vi "JOG LIMIT.vi"(8 "error in (no error)":errorcluster, 11 "main ref":T1) -> (0 "error out":errorcluster)   [LabVIEW 2025]
uses:
  controls/LAB-IQ UI Data.ctl
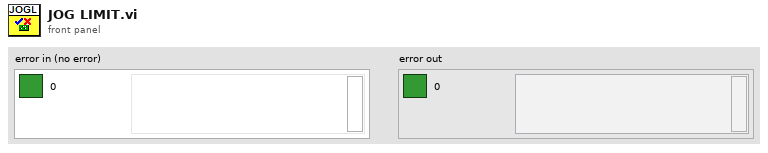
[diagram p1: front panel]
types:
  T1 = typedef "LAB-IQ UI Data.ctl" = cluster{"Main Home Screen":cluster{"GUI":refnum<vi>, "Platform Settings":refnum<vi>, "Configure":refnum<vi>, "Home":refnum<vi>, "EXIT":refnum<vi>, "service 2":refnum<vi>, "MainPage":refnum<vi>, "Analysis":refnum<vi>}, "Platform Settings":cluster{"mm/s  Surge":refnum<vi>, "Update Surge Speed":refnum<vi>, "Drive Error":refnum<vi>, "Disable Axis Jog Soft Limits":refnum<vi>, "mm/s  Sway":refnum<vi>, "Sway and Surge COM Status":refnum<vi>, "Heave COM Status":refnum<vi>, "Enable Platform":refnum<vi>, "Surge Forward Main":refnum<vi>, "Sway Right Main":refnum<vi>, "Sway Left Main":refnum<vi>, "Heave Down Main":refnum<vi>, "Heave Up main":refnum<vi>, "Update Sway Speed":refnum<vi>, "Update Heave Speed":refnum<vi>, "mm/s Heave":refnum<vi>, "mm/sec":refnum<vi>, "mm":refnum<vi>, "Surge Backward Main":refnum<vi>}, "Analysis Screen":cluster{"Analysis Home":refnum<vi>, "Surface Analysis":refnum<vi>, "Imaging":refnum<vi>, "Image Analysis":refnum<vi>, "Post Analysis":refnum<vi>}, "Config Screen":cluster{"Select Load Head":refnum<vi>, "Notes :":refnum<vi>, "FILE":refnum<vi>, "Sample ID :":refnum<vi>, "Operator ID :":refnum<vi>, "Operator Name :":refnum<vi>, "Auto":refnum<vi>}, "Motion Module":cluster{"zNL":refnum<vi>, "NL disp":refnum<vi>, "Rotary Tab":refnum<vi>, "Motion Direction:  3":refnum<vi>, "E.Velocity 2":refnum<vi>, "e.v/ssr 2":refnum<vi>, "Enter Fixed E.Velocity 2":refnum<vi>, "Enter Final SRR 2":refnum<vi>, "Enter initial SRR 2":refnum<vi>, "Enter Fixed SRR 2":refnum<vi>, "Enter the Final E.Velocity (m/s) 2":refnum<vi>, "Enter initial E.Velocity (m/s) 2":refnum<vi>, "Final Speed (RPM) 3":refnum<vi>, "Initial Speed (RPM) 2":refnum<vi>, "Enter the Final Velocity (m/s) 3":refnum<vi>, "Enter initial Velocity (m/s)  3":refnum<vi>, "Ramp Up 2":refnum<vi>, "TEST SELECTION":refnum<vi>, "SPEED SELECTION : ":refnum<vi>, "Angular Oscillation Set":refnum<vi>, "Traction":refnum<vi>, "Step Speed":refnum<vi>, "StepTable For Load-Speed":refnum<vi>, "StepTable For Speed":refnum<vi>, "Surge Forward MM":refnum<vi>, "Surge Backward MM":refnum<vi>, "M3 Image":refnum<vi>, "String 39":refnum<vi>, "Sway Left MM":refnum<vi>, "Sway Right MM":refnum<vi>, "Disable Axis Jog Soft Limits":refnum<vi>, "mm":refnum<vi>, "Heave Down MM":refnum<vi>, "Heave Up MM":refnum<vi>, "Wear Track Diameter (mm)":refnum<vi>, "Set WTD":refnum<vi>, "HomeScratch":refnum<vi>, "HomeRot":refnum<vi>, "PlaceModule":refnum<vi>, "Enter the Angle (Deg)":refnum<vi>, "Enter the Frequency (Hz)":refnum<vi>, "Motion Mode:":refnum<vi>, "LR Sway":refnum<vi>, "Rot Hor":refnum<vi>, "Scratch":refnum<vi>, "LR Cam":refnum<vi>, "MMBack":refnum<vi>, "MMNext":refnum<vi>, "Rot Ver":refnum<vi>, "Rotary Module Selection":refnum<vi>, "calculate rotary":refnum<vi>, "SPEED SELECTION : rotary":refnum<vi>, "Import 2":refnum<vi>, "Save 2":refnum<vi>, "File Path :  2":refnum<vi>, "String 45":refnum<vi>, "StepTable For Speed 3":refnum<vi>, "Enter the Speed(mm/sec)":refnum<vi>, "Enter the Speed(RPM)":refnum<vi>, "Enter Scratch Speed (mm/s):":refnum<vi>, "SwaySpeed Set":refnum<vi>, "Scartch Offset":refnum<vi>, "Motion type:":refnum<vi>, "HomeScratch 2":refnum<vi>, "Enter Scratch length (mm):":refnum<vi>, "Wear Track Diameter":refnum<vi>, "Rotary Speed Exced":refnum<vi>, "Scratch Mode":refnum<vi>, "No of Scratch":refnum<vi>}, "Environmental control":cluster{"Humidity  Status  3":refnum<vi>, "Low Temp  Status  2":refnum<vi>, "TK4 status 2":refnum<vi>, "Stage Temperature":refnum<vi>, "Sample Temperature":refnum<vi>, "Humidity (Amb)":refnum<vi>, "Clear List":refnum<vi>, "Add to list":refnum<vi>, "Wear":refnum<vi>, "Vibration":refnum<vi>, "Humidity (Chamber)":refnum<vi>, "Temperature (Chamber)":refnum<vi>, "ECR ":refnum<vi>, "Temperature (Amb)":refnum<vi>, "Microphone":refnum<vi>, "Acoustic Emission 3":refnum<vi>, "SNext":refnum<vi>, "APBack":refnum<vi>, "Enter the Temperature (°C):":refnum<vi>, "Enter the Stage \nTemperature (°C):":refnum<vi>, "Enter the Humidity (%Rh):":refnum<vi>, "Low Temp":refnum<vi>, "High Temp":refnum<vi>, "Humidity":refnum<vi>, "Sensors Picked":refnum<vi>}, "About Screen":cluster{"Password":refnum<vi>, "Home Service":refnum<vi>, "Advanced Setting":refnum<vi>, "About Tab":refnum<vi>, "ECR Port:":refnum<vi>, "Ramp Port:":refnum<vi>, "Installation/Replacement completed":refnum<vi>, "Loahead":refnum<vi>, "Heave and Surge COM Port:":refnum<vi>, "Sway COM Port:":refnum<vi>, "Temp Modbus:":refnum<vi>, "Humidity Port:":refnum<vi>, "Edit Gain Constants":refnum<vi>, "Save Gain Constants":refnum<vi>}, "Main Screen":cluster{"Main Screen Tab":refnum<vi>, "Angle and Frequency":refnum<vi>, "Stroke (mm)":refnum<vi>, "Angle (Deg)":refnum<vi>, "Main Speed Tab":refnum<vi>, "MTM MOTOR DISPLAY":refnum<vi>, "Disc Speed (m/sec)":refnum<vi>, "Ball Speed (m/sec)":refnum<vi>, "Disc Speed (RPM)":refnum<vi>, "Ball Speed (RPM)":refnum<vi>, "SPEED TAB":refnum<vi>, "Speed (m/sec)":refnum<vi>, "Set Speed (m/sec)":refnum<vi>, "Speed (RPM)":refnum<vi>, "Set Speed":refnum<vi>, "Time Tab":refnum<vi>, "Time ( HH:MM:SS ) 2":refnum<vi>, "Test Duration":refnum<vi>, "Test Duration 4":refnum<vi>, "TEST CYCLE":refnum<vi>, "TOTAL CYCLES":refnum<vi>, "Set Load (N)":refnum<vi>, "Temp Tabs":refnum<vi>, "Heater":refnum<vi>, "TK4 status":refnum<vi>, "ChamberTemp":refnum<vi>, "SetTmp":refnum<vi>, "Controller  Status":refnum<vi>, "ChamberTemp 2":refnum<vi>, "SetTmp 2":refnum<vi>, "Controller  Status 2":refnum<vi>, "ChamberTemp 3":refnum<vi>, "SetTmp 3":refnum<vi>, "Cooling":refnum<vi>, "Load Communication":refnum<vi>, "Ambient \nTemperature":refnum<vi>, "HumCOMStatus":refnum<vi>, "Ambient\n Humidity":refnum<vi>, "Freq (Hz)":refnum<vi>, "Load En":refnum<vi>, "NLt":refnum<vi>, "zNL 2":refnum<vi>, "Humidity On":refnum<vi>, "humidity disp":refnum<vi>, "Set Humidity":refnum<vi>, "NL disp 2":refnum<vi>, "Humidity On 2":refnum<vi>, "humidity disp 2":refnum<vi>, "Set Humidity 2":refnum<vi>, "NL disp 3":refnum<vi>, "AppLoadSeq scratch":refnum<vi>, "Stop Scratch":refnum<vi>, "ClrLog":refnum<vi>, "Trip Log":refnum<vi>, "STOP":refnum<vi>, "Start Test":refnum<vi>, "Test status":refnum<vi>, "AR Led":refnum<vi>, "Data":refnum<vi>, "Health":refnum<vi>, "Sway COM Status":refnum<vi>, "Heave COM Status":refnum<vi>, "Grp Tab":refnum<vi>, "Sub Graph":refnum<vi>, "SD (mm)":refnum<vi>, "Siliding distance Reset Graph":refnum<vi>, "SDGp":refnum<vi>, "Humidity Reset Graph":refnum<vi>, "HumrGp":refnum<vi>, "Acoustic Emission (mV)":refnum<vi>, "Aqucostic Reset Graph":refnum<vi>, "gACQUOS":refnum<vi>, "ECR RESET":refnum<vi>, "ECR":refnum<vi>, "Temperature Reset":refnum<vi>, "Acoustic Emission (mV) 2":refnum<vi>, "Aqucostic Reset Graph 2":refnum<vi>, "gACQUOS 2":refnum<vi>, "ECR RESET 2":refnum<vi>, "ECR 2":refnum<vi>, "Temperature Reset 2":refnum<vi>, "Temperature (deg c)":refnum<vi>, "Speed Reset Graph":refnum<vi>, "Speed Tab":refnum<vi>, "MTM DISC  SPEED":refnum<vi>, "MTM BALL SPEED":refnum<vi>, "speed mm/sec":refnum<vi>, "Hymidity":refnum<vi>, "Humidity Disable trip":refnum<vi>, "CoF Trip  2":refnum<vi>, "Depth Trip":refnum<vi>, "Weart Deapth":refnum<vi>, "Depth Reset Graph":refnum<vi>, "Weart":refnum<vi>, "Depthz":refnum<vi>, "Depth (µm)":refnum<vi>, "WearGp":refnum<vi>, "NL Trip 2":refnum<vi>, "Load pid":refnum<vi>, "Load Disable Trip":refnum<vi>, "Load Reset Graph":refnum<vi>, "NL Display 4":refnum<vi>, "Main Chart 3":refnum<vi>, "BACK":refnum<vi>, "Depth Trip 2":refnum<vi>, "COF TRIP ":refnum<vi>, "Friction Force (N)":refnum<vi>, "FF Reset Graph":refnum<vi>, "FF Disable Trip":refnum<vi>, "FF TRIP":refnum<vi>, "COF Disable Trip":refnum<vi>, "COF Reset Graph":refnum<vi>, "Start Test Temp":refnum<vi>, "zFF":refnum<vi>, "Friction Force (N) Graph":refnum<vi>, "Coefficient of Friction":refnum<vi>, "Scratch Start Test":refnum<vi>, "FF Tab":refnum<vi>, "Cyclic Friction Force (N)":refnum<vi>, "CZ FF":refnum<vi>, "Cyclic Friction Force (N) Graph":refnum<vi>, "Cyclic Coefficient of Friction":refnum<vi>, "Cyclic FF TRIP":refnum<vi>, "Cyclic FF Disable Trip":refnum<vi>, "cyclic COF Disable Trip":refnum<vi>, "cyclic COF TRIP":refnum<vi>, "cyclic COF Reset Graph":refnum<vi>, "Cyclic FF Reset Graph":refnum<vi>, "Test Trip":refnum<vi>, "Multi Scratch Pass":refnum<vi>, "Scratch Start Recording":refnum<vi>}, "Loading":cluster{"Indentation":refnum<vi>, "Reference Sample":refnum<vi>, "Load Cell Communication Slide":refnum<vi>, "com 3":refnum<vi>, "com":refnum<vi>, "DecaForce COM Status":refnum<vi>, "Update":refnum<vi>, "Clear 3":refnum<vi>, "seq":refnum<vi>, "Stribeck table":refnum<vi>, "Stribeck Table  For loading":refnum<vi>, "Loading Mode":refnum<vi>, "Enter the Final Load (N)":refnum<vi>, "Enter the CoF Trip":refnum<vi>, "Enter the Friction Force Trip":refnum<vi>, "Enter the Normal load Trip":refnum<vi>, "Enter the Load  (N)":refnum<vi>, "KiloForce":refnum<vi>, "DecaForce ":refnum<vi>, "MicroForce":refnum<vi>, "LHBack":refnum<vi>, "LHNext":refnum<vi>, "Enter the Loading Rate (N/min)":refnum<vi>, "Message":refnum<vi>, "Warning 2":refnum<vi>, "SSP 0.75":refnum<vi>, "SSP 0.5":refnum<vi>, "SSP 0.3":refnum<vi>, "Warning":refnum<vi>, "gui GIF":refnum<vi>, "Communication is established":refnum<vi>, "AppLoad 4":refnum<vi>, "Multipoint":refnum<vi>, "Load Selection":refnum<vi>}, "PID":cluster{"Ramp MulFac":refnum<vi>, "pulses LoadDiffRamp(2..10)":refnum<vi>, "PulseControlRamp(diff<=3N)":refnum<vi>, "SetLoadDeadband(%) Load(0-10N)":refnum<vi>, "PID gains out delay (microForce)":refnum<vi>, "Ramp":refnum<vi>, "Gain 2":refnum<vi>, "pulses LoadDiff(2..10)":refnum<vi>, "pulses LoadDiff(11..50)":refnum<vi>, "PulseControl(diff<=3N)":refnum<vi>, "SetLoadDeadband(%)  2":refnum<vi>, "Dummy Run":refnum<vi>, "Vertical load (N)":refnum<vi>, "AutoTune":refnum<vi>, "Offset 3 ":refnum<vi>, "apply load":refnum<vi>, "Offset  3":refnum<vi>, "apply load 2":refnum<vi>, "Enter ByPass Load":refnum<vi>, "reinit 3":refnum<vi>, "output range delay":refnum<vi>, "PID gains out delay":refnum<vi>, "Bypass Load":refnum<vi>, "pulsesSent":refnum<vi>, "pulses ":refnum<vi>, "actpid":refnum<vi>, "gFF Rot":refnum<vi>, "pulses LoadDiff(21..1000)":refnum<vi>, "Delay":refnum<vi>, "deadband":refnum<vi>}, "Config Parameters":cluster{"Tab Control 3":refnum<vi>, "Tab Control 19":refnum<vi>, "SAMPLES":refnum<vi>, "Re-initilaize":refnum<vi>, "Filter ON/OFF":refnum<vi>, "TracHomeSurgeOffsetCounts 10MM":refnum<vi>, "TracHomeSwayOffsetCounts 10MM":refnum<vi>, "Acoustic Emission:":refnum<vi>, "Apply Filter (FF)":refnum<vi>, "Filter% 2":refnum<vi>, "Apply Filter (Load)":refnum<vi>, "Filter% ":refnum<vi>, "Sway distance (mm)":refnum<vi>, "Surge distance (mm)":refnum<vi>, "DataSavingLoopDelay(ms)":refnum<vi>, "SAVE 2":refnum<vi>, "Enter Distance":refnum<vi>, "Sway Counts:":refnum<vi>, "Distance (mm): 3":refnum<vi>, "Surge Counts:":refnum<vi>, "Distance (mm): 2":refnum<vi>, "Distance (mm):":refnum<vi>, "Heave Counts:":refnum<vi>, "LRMHomeSurgeOffsetCounts":refnum<vi>, "LRMHomeSwayOffsetCounts":refnum<vi>, "TracHomeSurgeOffsetCounts 20MM":refnum<vi>, "TracHomeSwayOffsetCounts 20MM":refnum<vi>, "RotHomeSwayOffsetCounts":refnum<vi>, "RotHomeSurgeOffsetCounts":refnum<vi>, "Heave distance":refnum<vi>, "Zmm":refnum<vi>, "Heave Pulses/mm":refnum<vi>, "Surge Pulses/mm":refnum<vi>, "Sway Pulses/mm":refnum<vi>, "Heave Pitch":refnum<vi>, "Surge Pitch":refnum<vi>, "Sway Pitch":refnum<vi>, "Heave PPR":refnum<vi>, "Surge PPR":refnum<vi>, "Sway PPR":refnum<vi>, "Tab Control 5":refnum<vi>, "Tab Control 14":refnum<vi>, "Tab Control 26":refnum<vi>, "AE":refnum<vi>, "Heave Loop Delay":refnum<vi>, "Heave PID Speed":refnum<vi>, "Surge Jog Speed":refnum<vi>, "Heave Jog Speed":refnum<vi>, "Sway Loop Delay":refnum<vi>, "Sway PID Speed":refnum<vi>, "Sway Jog Speed":refnum<vi>, "DEPTH TRIP VALUE":refnum<vi>, "LOAD TRIP VALUE":refnum<vi>, "DEPTH TRIP   ENABLE":refnum<vi>, "LOAD TRIP  ENABLE":refnum<vi>, "CYCLIC FF TRIP VALUE":refnum<vi>, "FF TRIP VALUE":refnum<vi>, "CYCLIC CoF TRIP VALUE":refnum<vi>, "COF TRIP VALUE":refnum<vi>, "CYCLIC COF TRIP  ENABLE":refnum<vi>, "CYCLIC FF TRIP  ENABLE":refnum<vi>, "FF TRIP  ENABLE":refnum<vi>, "COF TRIP  ENABLE":refnum<vi>}, "Loading Com Port":cluster{"ClearAll":refnum<vi>, "Mz(Nm)":refnum<vi>, "My(Nm)":refnum<vi>, "Mx(Nm)":refnum<vi>, "Save Dwell":refnum<vi>, "Mx ":refnum<vi>, "My ":refnum<vi>, "Mz":refnum<vi>, "Fx(N)":refnum<vi>, "Fy(N)":refnum<vi>, "Fz(N)":refnum<vi>, "ZeroAll":refnum<vi>, "Acq Delay (ms)":refnum<vi>, "Burst Delay (ms)":refnum<vi>, "model":refnum<vi>, "SN":refnum<vi>, "FFx(N)":refnum<vi>, "Sensor IP":refnum<vi>, "Port":refnum<vi>, "FFy(N)":refnum<vi>, "Load(N)":refnum<vi>, "delete Handle":refnum<vi>, "Create Handle":refnum<vi>, "ft_data":refnum<vi>, "ft_range":refnum<vi>, "ft_data 2":refnum<vi>, "stop 6":refnum<vi>, "running_flag":refnum<vi>, "ft_udp_handle":refnum<vi>, "get-data-return":refnum<vi>, "get-range-return":refnum<vi>, "zero-return":refnum<vi>, "filter-return":refnum<vi>, "initial-return":refnum<vi>, "deleteHandle-result":refnum<vi>, "Load Cell Temp":refnum<vi>}, "Heave AND Surge":cluster{"SURGE POSE":refnum<vi>, "error out Read":refnum<vi>, "HEAVE POSE":refnum<vi>, "State":refnum<vi>, "Homed":refnum<vi>, "Sequence ID":refnum<vi>, "error out Write":refnum<vi>, "faultCode":refnum<vi>, "Ack ID":refnum<vi>, "SPEED":refnum<vi>, "Distance":refnum<vi>, "Mode Command":refnum<vi>, "Heave and Surge Read":refnum<vi>, "Read Heave Temp":refnum<vi>, "Spare 15":refnum<vi>, "Spare 14":refnum<vi>, "Spare 13":refnum<vi>, "Spare 12":refnum<vi>, "Spare 11":refnum<vi>, "Spare 10":refnum<vi>, "Spare 9":refnum<vi>, "Spare 8":refnum<vi>, "Spare 7":refnum<vi>, "Spare 6":refnum<vi>, "Spare 5":refnum<vi>, "Spare 4":refnum<vi>, "Spare 2":refnum<vi>, "Spare 1":refnum<vi>, "Node Id":refnum<vi>, "Spare 3":refnum<vi>, "SPARE 4":refnum<vi>, "SPARE 3":refnum<vi>, "SPARE 2":refnum<vi>, "SPARE 1":refnum<vi>, "fwMajor":refnum<vi>, "fwMinor":refnum<vi>, "Manual Write":refnum<vi>, "Heave and Surge Write":refnum<vi>}, "New PID LOGIC":cluster{"Fine Tune Zone":refnum<vi>, "PID SDelay":refnum<vi>, "Max_pos_limit":refnum<vi>, "Min_pos_limit":refnum<vi>, "i_limit":refnum<vi>, "pct_scale":refnum<vi>, "Deadband":refnum<vi>, "Kd":refnum<vi>, "Ki":refnum<vi>, "Kp":refnum<vi>, "Current Position":refnum<vi>, "Set Load":refnum<vi>, "Current Load":refnum<vi>, "Pulse delta":refnum<vi>, "Init Step":refnum<vi>, "Max Step Linit":refnum<vi>}, "SWAY ":cluster{"fwMajor":refnum<vi>, "Homed":refnum<vi>, "Rotary POSE":refnum<vi>, "State":refnum<vi>, "SWAY POSE":refnum<vi>, "Ack ID":refnum<vi>, "faultCode":refnum<vi>, "Node Id":refnum<vi>, "fwMinor":refnum<vi>, "Spare 6":refnum<vi>, "Spare 5":refnum<vi>, "Spare 4":refnum<vi>, "Spare 3":refnum<vi>, "Spare 2":refnum<vi>, "Spare 1":refnum<vi>, "Spare 7":refnum<vi>, "SPARE  5":refnum<vi>, "error out Write  SWAY ":refnum<vi>, "error out Read SWAY ":refnum<vi>, "Manual Write SWAY ":refnum<vi>, "SWAY WRITE":refnum<vi>, "SPARE  4":refnum<vi>, "SPARE  3":refnum<vi>, "SPARE 2":refnum<vi>, "SPARE 1":refnum<vi>, "Spare 15":refnum<vi>, "Spare 14":refnum<vi>, "Spare 13":refnum<vi>, "Spare 12":refnum<vi>, "Spare 11":refnum<vi>, "Spare 9":refnum<vi>, "Spare 8":refnum<vi>, "SPEED":refnum<vi>, "Distance":refnum<vi>, "Mode Command":refnum<vi>, "Sequence ID":refnum<vi>, "SWAY READ":refnum<vi>, "Spare 10":refnum<vi>, "Read SWAY Temp":refnum<vi>}, "Analysis Screen":cluster{"Analysis Home":refnum<vi>, "Refresh 2":refnum<vi>, "MEAN 4":refnum<vi>, "SD 4":refnum<vi>, "VARIANCE 4":refnum<vi>, "MEAN  3":refnum<vi>, "SD  3":refnum<vi>, "VARIANCE  3":refnum<vi>, "MEAN 2":refnum<vi>, "SD  2":refnum<vi>, "VARIANCE 2":refnum<vi>, "MEAN":refnum<vi>, "SD":refnum<vi>, "VARIANCE":refnum<vi>, "File 4 Discription":refnum<vi>, "OPEN 4":refnum<vi>, "File Name 4":refnum<vi>, "OPEN 3":refnum<vi>, "File 3 Discription":refnum<vi>, "File Name 3":refnum<vi>, "Y-AXIS":refnum<vi>, "X-AXIS":refnum<vi>, "XY Graph":refnum<vi>, "File Name 2":refnum<vi>, "File Name 1":refnum<vi>, "OPEN 2":refnum<vi>, "OPEN 1":refnum<vi>, "File 1 Discription ":refnum<vi>, "File 2 Discription":refnum<vi>, "Export":refnum<vi>, "File Format":refnum<vi>}}
  T2 = enum8{"Enabled", "Disabled", "Disabled and Grayed Out"}
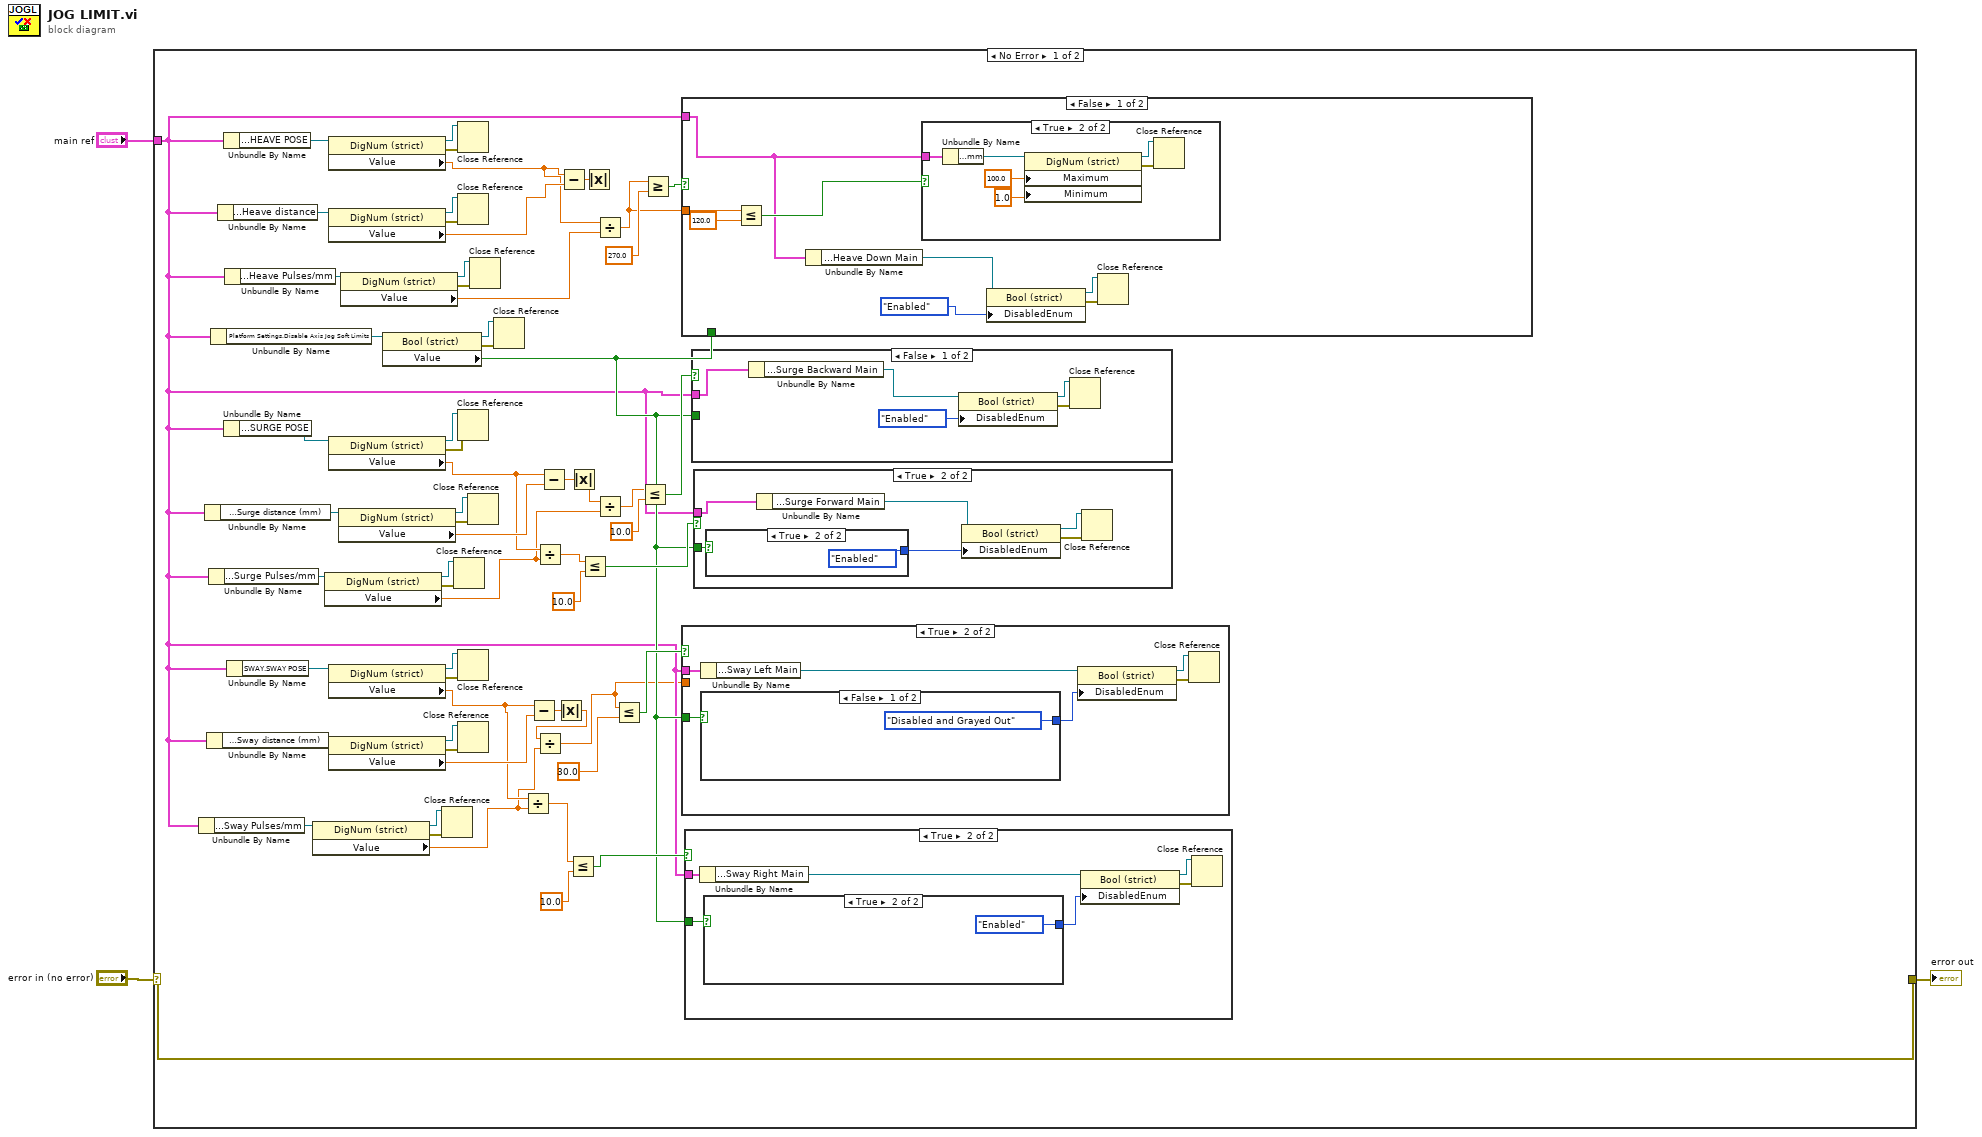
[diagram p0: block diagram]
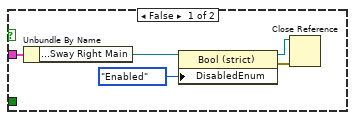
[diagram p2: hidden frame]
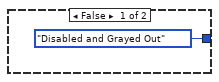
[diagram p3: hidden frame]
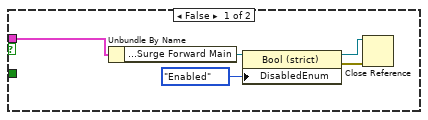
[diagram p4: hidden frame]
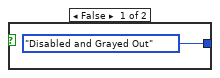
[diagram p5: hidden frame]
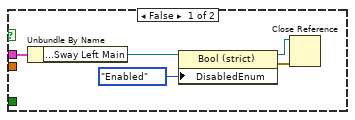
[diagram p6: hidden frame]
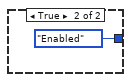
[diagram p7: hidden frame]
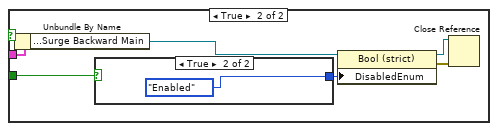
[diagram p8: hidden frame]
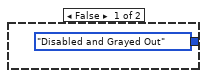
[diagram p9: hidden frame]
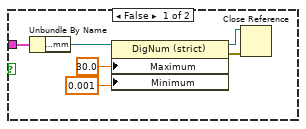
[diagram p10: hidden frame]
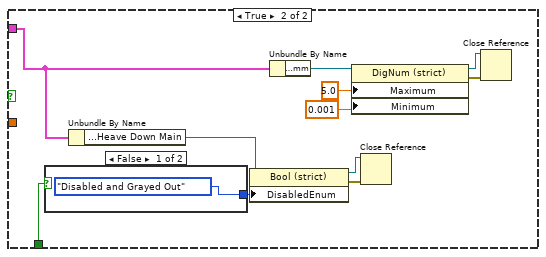
[diagram p11: hidden frame]
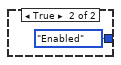
[diagram p12: hidden frame]
diagram:
  n1 = case shown="No Error" "error in (no error)" {
    selector: "error in (no error)" -> [w65 _]
    tunnel: [w65 _] -> w2
    tunnel: "main ref" -> [w13 _]
    frame No Error {
      n2 = Unbundle By Name(w13) -> ("Config Parameters.Sway Pulses/mm"=w28:refnum<vi>)
      n3 = Unbundle By Name(w13) -> ("Config Parameters.Surge distance (mm)"=w49:refnum<vi>)
      n4 = Unbundle By Name(w13) -> ("Config Parameters.Sway distance (mm)"=w44:refnum<vi>)
      n5 = Unbundle By Name(w13) -> ("Config Parameters.Surge Pulses/mm"=w36:refnum<vi>)
      n6 = Unbundle By Name(w13) -> ("Platform Settings.Disable Axis Jog Soft Limits"=w31:refnum<vi>)
      n7 = Unbundle By Name(w13) -> ("Config Parameters.Heave distance"=w62:refnum<vi>)
      n8 = Unbundle By Name(w13) -> ("Heave AND Surge.HEAVE POSE"=w61:refnum<vi>)
      n9 = Unbundle By Name(w13) -> ("Heave AND Surge.SURGE POSE"=w50:refnum<vi>)
      n10 = Unbundle By Name(w13) -> ("Config Parameters.Heave Pulses/mm"=w16:refnum<vi>)
      n11 = Unbundle By Name(w13) -> ("SWAY.SWAY POSE"=w43:refnum<vi>)
      n12 = property class="DigNum (strict)"(reference=w28) -> (reference out=w26:refnum<vi>, error out=w27:errorcluster, "Value"=w6:dbl)  [unwired: 1 in]
      n13 = property class="DigNum (strict)"(reference=w36) -> (reference out=w34:refnum<vi>, error out=w35:errorcluster, "Value"=w10:dbl)  [unwired: 1 in]
      n14 = property class="DigNum (strict)"(reference=w61) -> (reference out=w59:refnum<vi>, error out=w60:errorcluster, "Value"=w5:sgl)  [unwired: 1 in]
      n15 = property class="DigNum (strict)"(reference=w62) -> (reference out=w64:refnum<vi>, error out=w63:errorcluster, "Value"=w21:dbl)  [unwired: 1 in]
      n16 = property class="DigNum (strict)"(reference=w50) -> (reference out=w52:refnum<vi>, error out=w51:errorcluster, "Value"=w19:sgl)  [unwired: 1 in]
      n17 = property class="DigNum (strict)"(reference=w43) -> (reference out=w41:refnum<vi>, error out=w42:errorcluster, "Value"=w17:sgl)  [unwired: 1 in]
      n18 = property class="DigNum (strict)"(reference=w44) -> (reference out=w46:refnum<vi>, error out=w45:errorcluster, "Value"=w18:dbl)  [unwired: 1 in]
      n19 = property class="DigNum (strict)"(reference=w49) -> (reference out=w47:refnum<vi>, error out=w48:errorcluster, "Value"=w20:dbl)  [unwired: 1 in]
      n20 = property class="DigNum (strict)"(reference=w16) -> (reference out=w14:refnum<vi>, error out=w15:errorcluster, "Value"=w12:dbl)  [unwired: 1 in]
      n21 = property class="Bool (strict)"(reference=w31) -> (reference out=w29:refnum<vi>, error out=w30:errorcluster, "Value"=w22:bool)  [unwired: 1 in]
      n22 = Close Reference(reference=w26, error in (no error)=w27) -> ()  [unwired: 1 out]
      n23 = Close Reference(reference=w34, error in (no error)=w35) -> ()  [unwired: 1 out]
      n24 = Close Reference(reference=w59, error in (no error)=w60) -> ()  [unwired: 1 out]
      n25 = Close Reference(reference=w64, error in (no error)=w63) -> ()  [unwired: 1 out]
      n26 = Close Reference(reference=w52, error in (no error)=w51) -> ()  [unwired: 1 out]
      n27 = Close Reference(reference=w41, error in (no error)=w42) -> ()  [unwired: 1 out]
      n28 = Close Reference(reference=w46, error in (no error)=w45) -> ()  [unwired: 1 out]
      n29 = Close Reference(reference=w47, error in (no error)=w48) -> ()  [unwired: 1 out]
      n30 = Close Reference(reference=w14, error in (no error)=w15) -> ()  [unwired: 1 out]
      n31 = Close Reference(reference=w29, error in (no error)=w30) -> ()  [unwired: 1 out]
      n32 = Divide(x=w17, y=w6) -> (x/y=w24:dbl)
      n33 = Subtract(x=w17, y=w18) -> (x-y=w38:dbl)
      n34 = Divide(x=w19, y=w10) -> (x/y=w33:dbl)
      n35 = Subtract(x=w19, y=w20) -> (x-y=w55:dbl)
      n36 = Absolute Value(x=w38) -> (abs(x)=w8:dbl)
      n37 = Divide(x=w8, y=w6) -> (x/y=w7:dbl)
      n38 = Subtract(x=w5, y=w21) -> (x-y=w56:dbl)
      n39 = Less Or Equal?(x=w24, y=10.0) -> (x <= y?=w23:bool)
      n40 = Absolute Value(x=w55) -> (abs(x)=w11:dbl)
      n41 = Less Or Equal?(x=w33, y=10.0) -> (x <= y?=w32:bool)
      n42 = Absolute Value(x=w56) -> ()  [unwired: 1 out]
      n43 = Divide(x=w5, y=w12) -> (x/y=w4:dbl)
      n44 = Divide(x=w11, y=w10) -> (x/y=w9:dbl)
      n45 = Less Or Equal?(x=w7, y=30.0) -> (x <= y?=w39:bool)
      n46 = Less Or Equal?(x=w9, y=10.0) -> (x <= y?=w54:bool)
      n47 = Greater Or Equal?(x=w4, y=270.0) -> (x >= y?=w57:bool)
      n48 = case shown="False" w57 {
        tunnel: w13 -> [w119 w139]
        tunnel: w4 -> [w125 _]
        tunnel: w22 -> [_ w138]
        frame False {
          n49 = Less Or Equal?(x=w125, y=120.0) -> (x <= y?=w123:bool)
          n50 = Unbundle By Name(w119) -> ("Platform Settings.Heave Down Main"=w120:refnum<vi>)
          n51 = case shown="True" w123 {
            tunnel: w119 -> [w126 w132]
            frame False {
              n52 = Unbundle By Name(w126) -> ("Platform Settings.mm"=w131:refnum<vi>)
              n53 = property class="DigNum (strict)"(reference=w131, "Maximum"=30.0 ("Data Entry Limits:Maximum"), "Minimum"=0.001 ("Data Entry Limits:Minimum")) -> (reference out=w129:refnum<vi>, error out=w130:errorcluster)  [unwired: 1 in]
              n54 = Close Reference(reference=w129, error in (no error)=w130) -> ()  [unwired: 1 out]
            }
            frame True {
              n55 = Unbundle By Name(w132) -> ("Platform Settings.mm"=w137:refnum<vi>)
              n56 = property class="DigNum (strict)"(reference=w137, "Maximum"=100.0 ("Data Entry Limits:Maximum"), "Minimum"=1.0 ("Data Entry Limits:Minimum")) -> (reference out=w135:refnum<vi>, error out=w136:errorcluster)  [unwired: 1 in]
              n57 = Close Reference(reference=w135, error in (no error)=w136) -> ()  [unwired: 1 out]
            }
          }
          n58 = property class="Bool (strict)"(reference=w120, "DisabledEnum"=T2."Enabled" ("Disabled")) -> (reference out=w122:refnum<vi>, error out=w121:errorcluster)  [unwired: 1 in]
          n59 = Close Reference(reference=w122, error in (no error)=w121) -> ()  [unwired: 1 out]
        }
        frame True {
          n60 = case shown="False" w138 {
            tunnel: [T2."Disabled and Grayed Out" ("Disabled") T2."Enabled" ("Disabled")] -> w143
            frame False {
            }
            frame True {
            }
          }
          n61 = Unbundle By Name(w139) -> ("Platform Settings.Heave Down Main"=w140:refnum<vi>)
          n62 = property class="Bool (strict)"(reference=w140, "DisabledEnum"=w143) -> (reference out=w142:refnum<vi>, error out=w141:errorcluster)  [unwired: 1 in]
          n63 = Unbundle By Name(w139) -> ("Platform Settings.mm"=w148:refnum<vi>)
          n64 = property class="DigNum (strict)"(reference=w148, "Maximum"=5.0 ("Data Entry Limits:Maximum"), "Minimum"=0.001 ("Data Entry Limits:Minimum")) -> (reference out=w146:refnum<vi>, error out=w147:errorcluster)  [unwired: 1 in]
          n65 = Close Reference(reference=w142, error in (no error)=w141) -> ()  [unwired: 1 out]
          n66 = Close Reference(reference=w146, error in (no error)=w147) -> ()  [unwired: 1 out]
        }
      }
      n67 = case shown="True" w39 {
        tunnel: w13 -> [w93 w98]
        tunnel: w7 -> [_ _]
        tunnel: w22 -> [_ w97]
        frame False {
          n68 = Unbundle By Name(w93) -> ("Platform Settings.Sway Left Main"=w96:refnum<vi>)
          n69 = property class="Bool (strict)"(reference=w96, "DisabledEnum"=T2."Enabled" ("Disabled")) -> (reference out=w94:refnum<vi>, error out=w95:errorcluster)  [unwired: 1 in]
          n70 = Close Reference(reference=w94, error in (no error)=w95) -> ()  [unwired: 1 out]
        }
        frame True {
          n71 = Unbundle By Name(w98) -> ("Platform Settings.Sway Left Main"=w102:refnum<vi>)
          n72 = case shown="False" w97 {
            tunnel: [T2."Disabled and Grayed Out" ("Disabled") T2."Enabled" ("Disabled")] -> w99
            frame False {
            }
            frame True {
            }
          }
          n73 = property class="Bool (strict)"(reference=w102, "DisabledEnum"=w99) -> (reference out=w100:refnum<vi>, error out=w101:errorcluster)  [unwired: 1 in]
          n74 = Close Reference(reference=w100, error in (no error)=w101) -> ()  [unwired: 1 out]
        }
      }
      n75 = case shown="True" w23 {
        tunnel: w13 -> [w67 w72]
        tunnel: w22 -> [_ w71]
        frame False {
          n76 = Unbundle By Name(w67) -> ("Platform Settings.Sway Right Main"=w70:refnum<vi>)
          n77 = property class="Bool (strict)"(reference=w70, "DisabledEnum"=T2."Enabled" ("Disabled")) -> (reference out=w68:refnum<vi>, error out=w69:errorcluster)  [unwired: 1 in]
          n78 = Close Reference(reference=w68, error in (no error)=w69) -> ()  [unwired: 1 out]
        }
        frame True {
          n79 = Unbundle By Name(w72) -> ("Platform Settings.Sway Right Main"=w76:refnum<vi>)
          n80 = case shown="True" w71 {
            tunnel: [T2."Disabled and Grayed Out" ("Disabled") T2."Enabled" ("Disabled")] -> w73
            frame False {
            }
            frame True {
            }
          }
          n81 = property class="Bool (strict)"(reference=w76, "DisabledEnum"=w73) -> (reference out=w74:refnum<vi>, error out=w75:errorcluster)  [unwired: 1 in]
          n82 = Close Reference(reference=w74, error in (no error)=w75) -> ()  [unwired: 1 out]
        }
      }
      n83 = case shown="False" w54 {
        tunnel: w13 -> [w105 w111]
        tunnel: w22 -> [_ w110]
        frame False {
          n84 = Unbundle By Name(w105) -> ("Platform Settings.Surge Backward Main"=w109:refnum<vi>)
          n85 = property class="Bool (strict)"(reference=w109, "DisabledEnum"=T2."Enabled" ("Disabled")) -> (reference out=w107:refnum<vi>, error out=w108:errorcluster)  [unwired: 1 in]
          n86 = Close Reference(reference=w107, error in (no error)=w108) -> ()  [unwired: 1 out]
        }
        frame True {
          n87 = Unbundle By Name(w111) -> ("Platform Settings.Surge Backward Main"=w115:refnum<vi>)
          n88 = case shown="True" w110 {
            tunnel: [T2."Disabled and Grayed Out" ("Disabled") T2."Enabled" ("Disabled")] -> w112
            frame False {
            }
            frame True {
            }
          }
          n89 = property class="Bool (strict)"(reference=w115, "DisabledEnum"=w112) -> (reference out=w113:refnum<vi>, error out=w114:errorcluster)  [unwired: 1 in]
          n90 = Close Reference(reference=w113, error in (no error)=w114) -> ()  [unwired: 1 out]
        }
      }
      n91 = case shown="True" w32 {
        tunnel: w13 -> [w79 w85]
        tunnel: w22 -> [_ w84]
        frame False {
          n92 = Unbundle By Name(w79) -> ("Platform Settings.Surge Forward Main"=w83:refnum<vi>)
          n93 = property class="Bool (strict)"(reference=w83, "DisabledEnum"=T2."Enabled" ("Disabled")) -> (reference out=w81:refnum<vi>, error out=w82:errorcluster)  [unwired: 1 in]
          n94 = Close Reference(reference=w81, error in (no error)=w82) -> ()  [unwired: 1 out]
        }
        frame True {
          n95 = case shown="True" w84 {
            tunnel: [T2."Disabled and Grayed Out" ("Disabled") T2."Enabled" ("Disabled")] -> w86
            frame False {
            }
            frame True {
            }
          }
          n96 = Unbundle By Name(w85) -> ("Platform Settings.Surge Forward Main"=w89:refnum<vi>)
          n97 = property class="Bool (strict)"(reference=w89, "DisabledEnum"=w86) -> (reference out=w87:refnum<vi>, error out=w88:errorcluster)  [unwired: 1 in]
          n98 = Close Reference(reference=w87, error in (no error)=w88) -> ()  [unwired: 1 out]
        }
      }
    }
    frame Error {
    }
  }
  "error out" <- w2
